vi "SetSplitWireIfLongDistance.vi"(0 "reference":refnum<class "SegmentedLineEdge.lvclass">, 2 "MaxLength":dbl=180.0, 5 "error in (no error)":errorcluster) -> (14 "reference out":refnum<class "SegmentedLineEdge.lvclass">, 19 "error out":errorcluster)   [LabVIEW 2014, in "SegmentedLineEdge.lvclass"]
doc: "public void draw(Graphics2D g2)"
uses:
  <resource>/Framework/Providers/Open_GDS/UML/SegmentedLineEdge_class/SegmentedLineEdge.lvclass
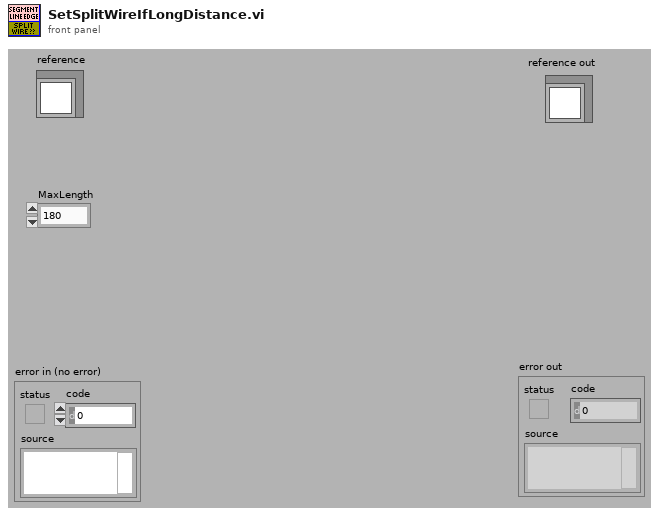
[diagram p1: front panel]
types:
  T1 = typedef "Point Point2D.ctl" = cluster{"x":dbl, "y":dbl}
  T2 = typedef "SegmentedLineEdge.lvclass/ObjectAttributes.ctl" = cluster{"lineStyle":refnum<class "LineStyle.lvclass">, "startArrowHead":refnum<class "ArrowHead.lvclass">, "endArrowHead":refnum<class "ArrowHead.lvclass">, "startLabel":string, "midLabel":string, "endLabel":string, "MidLabelOffset":T1, "SplitWire":bool}
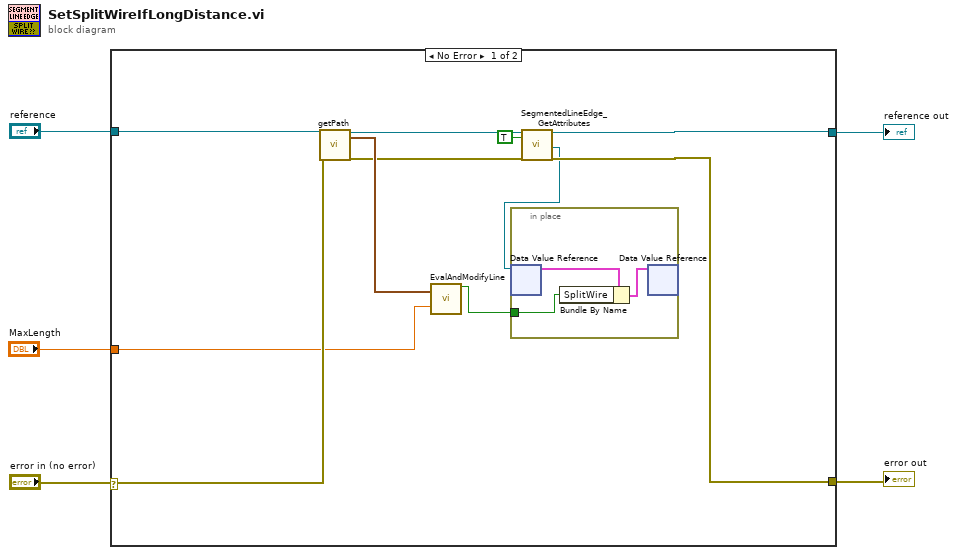
[diagram p0: block diagram]
diagram:
  n1 = case shown="No Error" "error in (no error)" {
    selector: "error in (no error)" -> [w15 w20]
    tunnel: "reference" -> [w13 w21]
    tunnel: [w10 w20] -> w4
    tunnel: [w9 w21] -> w3
    tunnel: "MaxLength" -> [w14 _]
    frame No Error {
      n2 = call-dynamic "getPath.vi"("reference"=w13, "error in (no error)"=w15) -> ("reference out"=w12:refnum<class "SegmentedLineEdge.lvclass">, "path"=w16:T1[], "error out"=w11:errorcluster)  [unwired: 15 in]
      n3 = call <resource>:"EvalAndModifyLine.vi"("path 2"=w16, "MaxLength"=w14) -> ("Ecxeeded"=w6:bool)  [unwired: 2 in, 15 out]
      n4 = call <resource>:"SegmentedLineEdge_GetAttributes.vi"("reference in"=w12, "OnlyGetDvrReference(False)"=TRUE, "error in (no error)"=w11) -> ("reference out"=w9:refnum<class "SegmentedLineEdge.lvclass">, "DataRef"=w7:refnum<data-value>, "error out"=w10:errorcluster)  [unwired: 13 in, 1 out]
      n5 = in-place {
        in-place-border: w6 -> [w18]
        n6 = in-place-dvr #1(w7) -> (w19:T2)  [unwired: 1 out]
        n7 = Bundle By Name(cluster=w19, "SplitWire"=w18) -> (w17:T2)
        n8 = in-place-dvr #1(w17) -> ()  [unwired: 2 out]
      }
    }
    frame Error {
    }
  }
  "reference out" <- w3
  "error out" <- w4
